vi "Get Addon Error Messges.vi"(8 "error in (no error)":errorcluster, 11 "Message Group in":u64) -> (0 "error out":errorcluster, 2 "Error Messages out":cluster{"Code":i32, "String":string}[](array[cluster]), 3 "Message Group out":u64)   [LabVIEW 2020, in "Instrument Addon Scripting API.lvlib"]
uses:
  Instrument Addon Scripting API.lvlib
  Shared Directory/FG Control.ctl
  <vilib>/NI VeriStand/Custom Device Tools/Custom Device Utility Library/Search Direction.ctl
  Shared Directory/Constants.vi
  <vilib>/NI VeriStand/Custom Device Tools/Custom Device Utility Library/NI VeriStand - Search for Item by GUID.vi
  Dependencies.llb/Instrument_Addon_Scripting_Dependencies_SysDef.Property.Get.vi
  Dependencies.llb/Instrument_Addon_Scripting_Dependencies_SysDef.Property.Get.String.vi
  Dependencies.llb/Instrument_Addon_Scripting_Dependencies_SysDef.Property.Set.vi
  Dependencies.llb/Instrument_Addon_Scripting_Dependencies_SysDef.Property.Set.String.vi
  <vilib>/Utility/LVClass/Get LV Class Default Value.vi
  Libraries Directory/Protocols.lvlibp/Protocol Parent/Protocol Parent.lvclass
  Shared Directory/Instrument Addon Shared.lvlib
  <vilib>/NI VeriStand/Custom Device Tools/Custom Device Utility Library/Custom Device Utility Library.lvlib
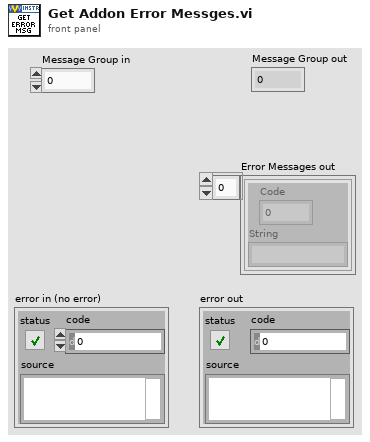
[diagram p1: front panel]
types:
  T1 = typedef "Instrument Addon Shared.lvlib/FG Control.ctl" = enum16{"Get", "Set"}
  T2 = typedef "Custom Device Utility Library.lvlib/Search Direction.ctl" = enum16{"Down", "Up"}
  T3 = typedef "Custom Device API.lvlib/Custom Device Item Ref.ctl" = u64
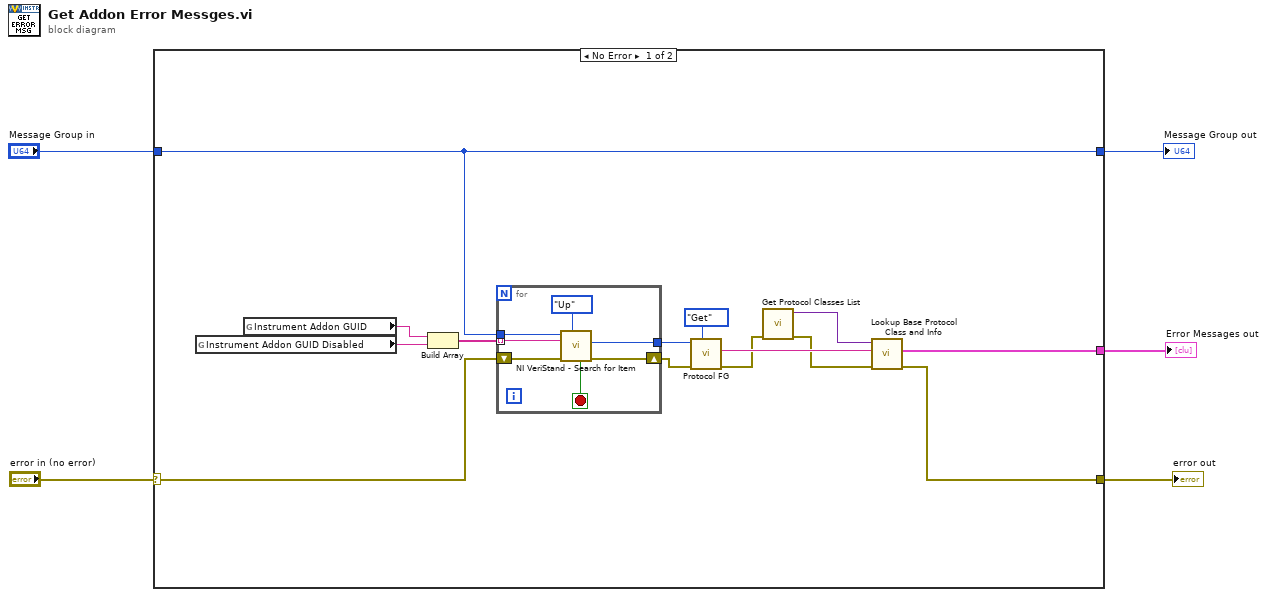
[diagram p0: block diagram]
diagram:
  n1 = case shown="No Error" "error in (no error)" {
    selector: "error in (no error)" -> [w7 w28]
    tunnel: "Message Group in" -> [w6 w27]
    tunnel: [w9 w28] -> w4
    tunnel: [w8 _] -> w3
    tunnel: [w6 w27] -> w1
    frame No Error {
      n2 = global read "Constants.vi" "Instrument Addon GUID Disabled"() -> (w17:string)
      n3 = global read "Constants.vi" "Instrument Addon GUID"() -> (w19:string)
      n4 = Build Array(w19, w17) -> (w18:string[])
      n5 = for {
        tunnel: w18 -> [w24] mode=indexing
        tunnel: [w22] -> w14
        shift-right: [w21] -> w10
        shift-left: w7 -> [w25]
        tunnel: w6 -> [w20]
        stop <- w23 stop-if-true
        n6 = call-poly <vilib>:"NI VeriStand - Search for Item.vi"("Direction (Down)"=Search_Direction."Up", "error in"=w25, "Item GUID"=w24, "Section Ref in"=w20) -> ("error out"=w21:errorcluster, "Item Ref"=w22:T3, "Found"=w23:bool)  [unwired: 4 in, 1 out]
      }
      n7 = call "Protocol FG.vi"("Action"=FG_Control."Get", "error in (no error)"=w10, "Device Item Ref in"=w14) -> ("error out"=w13:errorcluster, "Protocol out"=w15:string)  [unwired: 6 in, 1 out]
      n8 = call "Get Protocol Classes List.vi"("error in (no error)"=w13) -> ("error out"=w12:errorcluster, "Class Lookup"=w11:variant)  [unwired: 9 in]
      n9 = call "Lookup Base Protocol Class and Info.vi"("error in (no error)"=w12, "Protocol in"=w15, "Class Lookup"=w11) -> ("error out"=w9:errorcluster, "Error Codes"=w8:cluster{"Code":i32, "String":string}[])  [unwired: 4 in, 3 out]
    }
    frame Error {
    }
  }
  "Error Messages out" <- w3
  "error out" <- w4
  "Message Group out" <- w1
